vi "average.vi"(0 "JEC rCT001A":dbl, 1 "AO1":dbl, 2 "SI100 Avg Temp Rise":dbl, 3 "A-CON_DT_ACT_COR.Value":dbl, 4 "A-CON_ZP_ACT_COR.Value":dbl) -> (16 "ACT Loop":dbl)   [LabVIEW 2022 SP3, in "SI101.lvclass"]
uses:
  SI101.lvclass
  SI101.lvclass/SI101.ctl
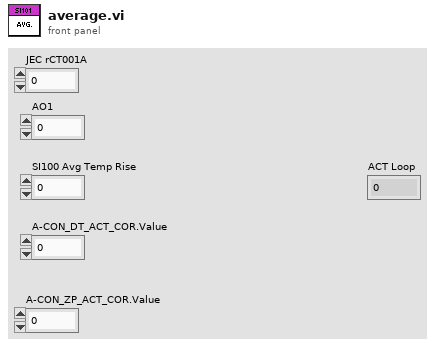
[diagram p1: front panel]
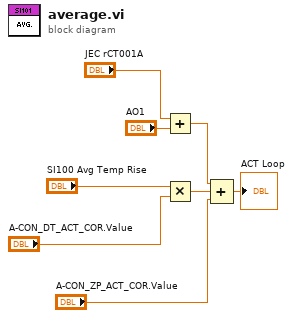
[diagram p0: block diagram]
diagram:
  n1 = Add(x="JEC rCT001A", y="AO1") -> (x+y=w4:dbl)
  n2 = Multiply(x="SI100 Avg Temp Rise", y="A-CON_DT_ACT_COR.Value") -> (x*y=w6:dbl)
  n3 = Compound Arithmetic op=ADD(w4, w6, "A-CON_ZP_ACT_COR.Value") -> (→"ACT Loop":dbl)
